vi "Update Pixel Signal.vi"(8 "error in (no error)":errorcluster, 9 "Cursor.Cursor Position":T1, 10 "Image Series":u16[](array[numeric]), 11 "Series Graph in":refnum<class "Series Graph.lvclass">) -> (0 "error out":errorcluster, 1 "Z Pixel Signal":u16[](array[numeric]), 3 "Series Graph out":refnum<class "Series Graph.lvclass">)   [LabVIEW 2023, in "Series Graph.lvclass"]
uses:
  Series Graph.lvclass
  D:/git/Graph-Classes/graph-classes/Base Graph/Base Graph.lvclass
  <vilib>/Utility/miscctls.llb/LVPointDoubleTypeDef.ctl
  Base Graph/Base Graph.lvclass/Base Graph.ctl
  Series Graph.lvclass/Series Graph.ctl
  Base Graph/Base Graph.lvclass
  D:/git/Graph-Classes/graph-classes/Detail Graph/Detail Graph.lvclass
  D:/git/Graph-Classes/graph-classes/Series Graph/Series Graph.lvclass
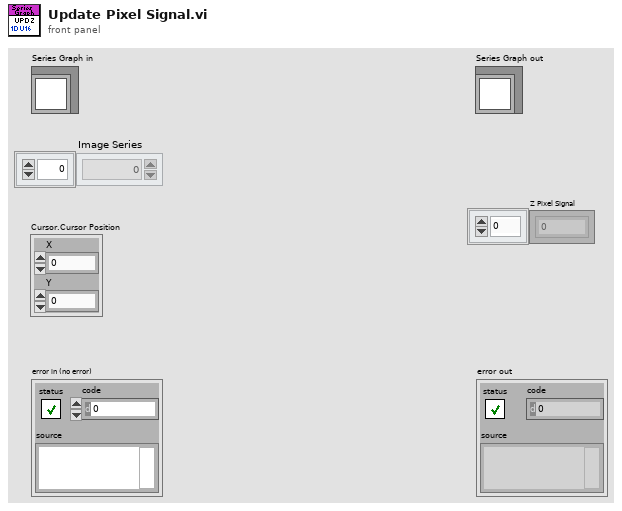
[diagram p1: front panel]
types:
  T1 = typedef "LVPointDoubleTypeDef.ctl" = cluster{"X":dbl, "Y":dbl}
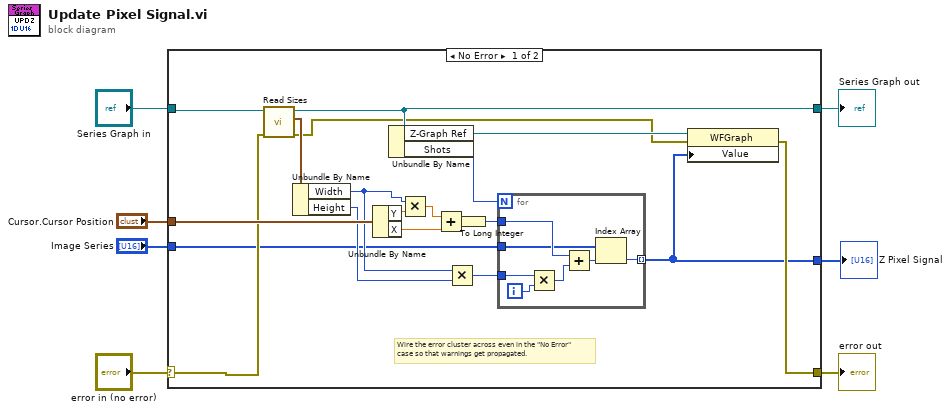
[diagram p0: block diagram]
diagram:
  n1 = case shown="No Error" "error in (no error)" {
    selector: "error in (no error)" -> [w15 w35]
    tunnel: [w19 w35] -> w6
    tunnel: [w16 w34] -> w4
    tunnel: "Series Graph in" -> [w17 w34]
    tunnel: "Cursor.Cursor Position" -> [w18 _]
    tunnel: "Image Series" -> [w9 _]
    tunnel: [w8 _] -> w1
    frame No Error {
      # "Wire the error cluster across even in the \"No Error\"\ncase so that warnings get propagated."
      n2 = call "Read Sizes.vi"("error in (no error)"=w15, "TG Base Graph in"=w17) -> ("error out"=w13:errorcluster, "Sizes"=w14:cluster{"Height":u32, "Width":u32}, "TG Base Graph out"=w16:refnum<class "Series Graph.lvclass">)  [unwired: 7 in]
      n3 = Unbundle By Name(w14) -> ("Width"=w11:u32, "Height"=w10:u32)
      n4 = Unbundle By Name(w18) -> ("Y"=w24:dbl, "X"=w26:dbl)
      n5 = Unbundle By Name(w16) -> ("Z-Graph Ref"=w20:refnum<vi>, "Shots"=w21:u32)
      n6 = Multiply(x=w11, y=w24) -> (x*y=w23:dbl)
      n7 = Add(x=w23, y=w26) -> (x+y=w25:dbl)
      n8 = Multiply(x=w11, y=w10) -> (x*y=w12:u32)
      n9 = To Long Integer(number=w25) -> (32bit integer=w22:i32)
      n10 = for {
        N: w21 -> [_]
        tunnel: w9 -> [w28]
        tunnel: w12 -> [w32]
        tunnel: w22 -> [w29]
        tunnel: [w27] -> w8 mode=indexing
        i -> [w33]
        n11 = Multiply(x=w32, y=w33) -> (x*y=w30:u32)
        n12 = Add(x=w29, y=w30) -> (x+y=w31:u32)
        n13 = Index Array(array=w28, index=w31) -> (element=w27:u16)
      }
      n14 = property class="WFGraph"(reference=w20, error in=w13, "Value"=w8) -> (error out=w19:errorcluster)  [unwired: 1 out]
    }
    frame Error {
    }
  }
  "error out" <- w6
  "Series Graph out" <- w4
  "Z Pixel Signal" <- w1
